vi "DestroyPrivateEvents.vi"(8 "error in (no error)":errorcluster, 11 "Inst.Krohn-Hite-7008":refnum<class "Inst.Krohn-Hite-7008.lvclass">) -> (0 "error out":errorcluster, 3 "Inst.Krohn-Hite-7008 out":refnum<class "Inst.Krohn-Hite-7008.lvclass">)   [LabVIEW 2019, in "Inst.Krohn-Hite-7008.lvclass"]
doc: "JKI State Machine Objects (SMO) 1.0.0.5\nJKI - JKI\nCopyright (c) 2016, JKI"
uses:
  Inst.Krohn-Hite-7008.lvclass
  <userlib>/LevyLab/Instrument Framework/Instrument Types/VSource/Instrument.VSource.lvclass
panel:
  # "For instructions on how to use the JKI State Machine Objects, examples and video tutorials, visit:\nhttp://jki.net/state-machine-objects/\n\nJKI State Machine Objects™\nhttp://jki.net/state-machine-objects/\nCopyright (C) 2005-2015, JKI <info@jki.net>\nALL RIGHTS RESERVED"
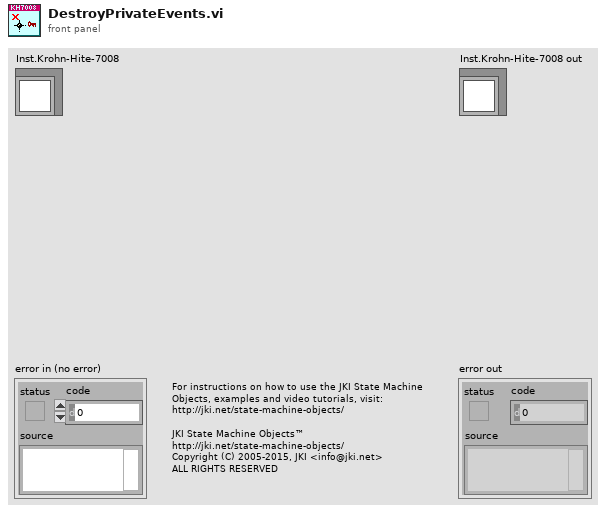
[diagram p1: front panel]
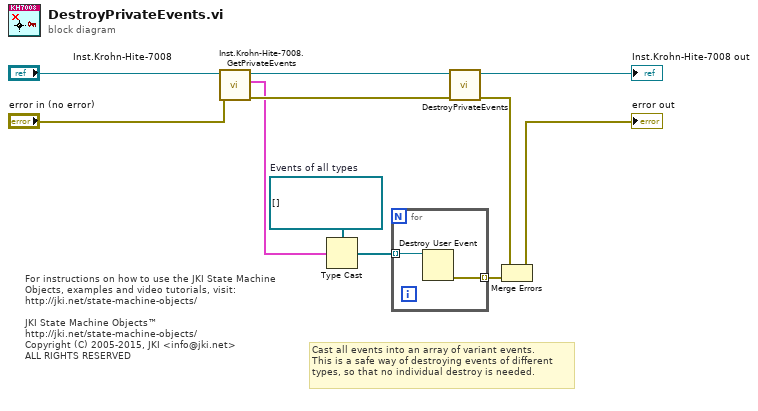
[diagram p0: block diagram]
diagram:
  w8 = refnum<user-event>[] []  # Events of all types
  # "For instructions on how to use the JKI State Machine Objects, examples and video tutorials, visit:\nhttp://jki.net/state-machine-objects/\n\nJKI State Machine Objects™\nhttp://jki.net/state-machine-objects/\nCopyright (C) 2005-2015, JKI <info@jki.net>\nALL RIGHTS RESERVED"
  # "Cast all events into an array of variant events.\nThis is a safe way of destroying events of different\ntypes, so that no individual destroy is needed."
  n1 = call "Inst.Krohn-Hite-7008.GetPrivateEvents.vi"("error in (no error)"="error in (no error)", "Inst.Krohn-Hite-7008 in"="Inst.Krohn-Hite-7008") -> ("error out"=w2:errorcluster, "Inst.Krohn-Hite-7008 Private Events"=w1:cluster{"MessageToProcess":refnum<user-event>}, "Inst.Krohn-Hite-7008 out"=w4:refnum<class "Inst.Krohn-Hite-7008.lvclass">)  [unwired: 7 in]
  n2 = Type Cast(type=w8, x=w1) -> (*(type *) &x=w9:refnum<user-event>[])
  n3 = for {
    tunnel: w9 -> [w13] mode=indexing
    tunnel: [w12] -> w7 mode=indexing
    n4 = Destroy User Event(user event=w13) -> (error out=w12:errorcluster)  [unwired: 1 in]
  }
  n5 = call-parent "DestroyPrivateEvents.vi"("error in (no error)"=w2, "Instrument"=w4) -> ("error out"=w5:errorcluster, "Instrument out"=→"Inst.Krohn-Hite-7008 out":refnum<class "Inst.Krohn-Hite-7008.lvclass">)  [unwired: 8 in]
  n6 = Merge Errors(w5, w7) -> (→"error out":errorcluster)
